vi "Get Software root and experiment.vi"(0 "Application in":refnum<vi>, 1 "This VI":refnum<vi>, 5 "Experiment name in":string, 7 "Sotware root in":string, 9 "FileVersion":string, 11 "error in":errorcluster) -> (3 "Yes?":bool, 4 "Numeric":i32, 6 "Mcast address":string, 10 "Sotware root out":string, 14 "Experiment namet":string, 15 "error out":errorcluster)   [LabVIEW 2020]
doc: "This vi find out experiment from arguments and get software root"
uses:
  Shared/MySQL/Preset Query Enum.ctl
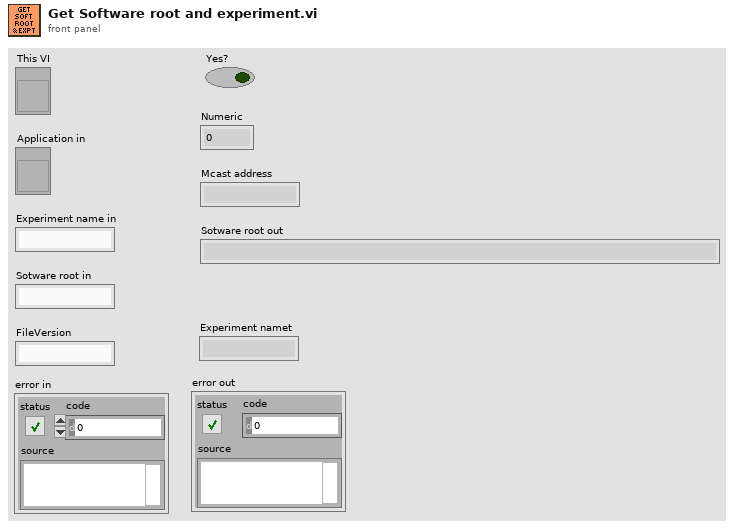
[diagram p1: front panel]
types:
  T1 = typedef "Preset Query Enum.ctl" = enum16{"Get Locations", "Get all IPs and MACs", "Get classes", "Get expt variables to set at scanstart for particular device", "Get expt devices and variables with start values", "Get expt devices and variables (with data to get)", "Get expt devices with data to get", "Get Expt devices and GUIs", "Get all devices basic properties", "Get Virtual Devices Core Info", "Get Expt names", "Get experiment basic properties", "Get experiment alarm variables", "Get MC Ports", "Get device network comm port", "Get devicetype lvclass path", "Get basic device properties", "Get Init Order", "Get all setable variables of a device", "Get device variable aliases", "Get force values of all settable variables", "Get all variables of a devicetype", "Get all variables of a device", "Get plotter details", "Get Saved Scans", "Get Scan Info", "GetGeneralGUIs", "Get expt for plotter", "Get plotter IDs from expt", "Get all devices", "Get all Virtual Devices", "Get all aliases", "Get variable and device info for Virtual Device", "GetItemLocatorIP", "Get IPs for GUIs", "Get DeviceType from Device", "GetLocalPortRange", "GetDevicePresetVariables", "Get Device Configuration", "GetAllPresetNames", "GetAllConfigurationNames", "GetPresetDeviceNames"}
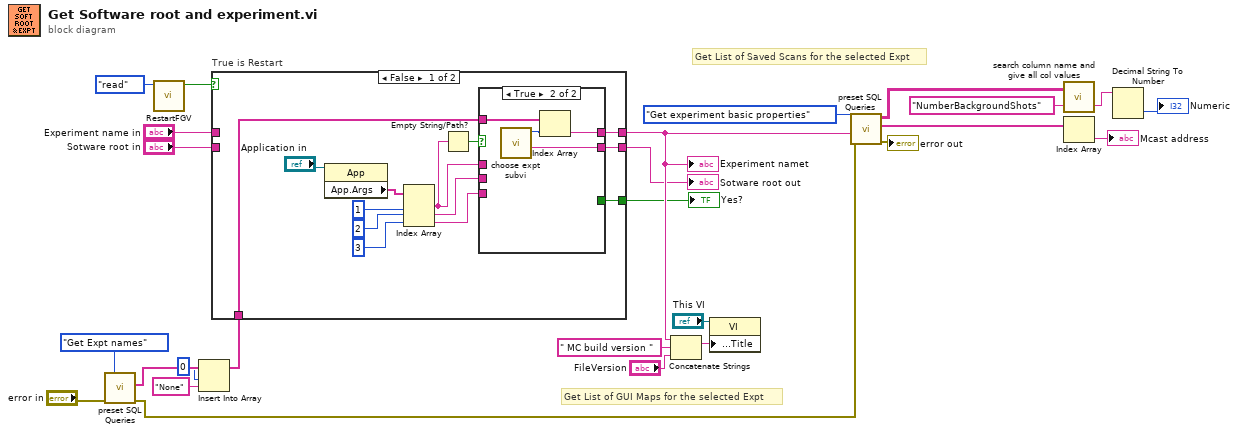
[diagram p0: block diagram]
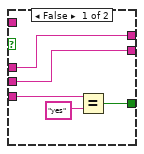
[diagram p2: hidden frame]
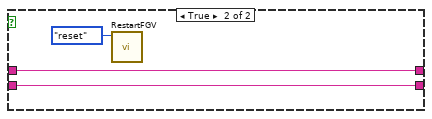
[diagram p3: hidden frame]
diagram:
  # "Get List of Saved Scans for the selected Expt"
  # "Get List of GUI Maps for the selected Expt"
  n1 = call "preset SQL Queries.vi"("error in (no error)"="error in", "Preset Query"=Preset_Query_Enum."Get Expt names") -> ("error out"=w1:errorcluster, "1st column 1st data"=w5:string[])  [unwired: 7 in, 1 out]
  n2 = call "RestartFGV.vi"("Function"=enum16{"set", "reset", "read"}."read") -> ("first call out"=w13:bool)  [unwired: 9 in, 1 out]
  n3 = Insert Into Array(array=w5, index=0, new element="None" ("new element/subarray")) -> (w7:string[])
  n4 = case "True is Restart" shown="False" w13 {
    tunnel: w7 -> [w39 _]
    tunnel: [w38 w50] -> w8
    tunnel: [w37 w51] -> w20
    tunnel: "Experiment name in" -> [_ w51]
    tunnel: "Sotware root in" -> [_ w50]
    tunnel: [w27 _] -> w19
    frame False {
      n5 = property class="App"(reference="Application in") -> ("App.Args"=w34:string[])  [unwired: 1 in, 2 out]
      n6 = Index Array(array=w34, index #1=1 ("index"), index #2=2 ("index"), index #3=3 ("index")) -> (element #1=w30:string, element #2=w31:string, element #3=w28:string)
      n7 = Empty String/Path?(string/path=w30) -> (empty?=w33:bool)
      n8 = case shown="True" w33 {
        tunnel: w39 -> [_ w47]
        tunnel: [w41 w46] -> w38
        tunnel: [w44 w45] -> w37
        tunnel: w31 -> [w41 _]
        tunnel: w30 -> [w44 _]
        tunnel: w28 -> [w40 _]
        tunnel: [w42 _] -> w27
        frame False {
          n9 = Equal?(x=w40, y="yes") -> (x = y?=w42:bool)
        }
        frame True {
          n10 = call "choose expt subvi.vi"() -> ("Software root"=w46:string, "Choosen\nExperiment out"=w48:u16)  [unwired: 10 in]
          n11 = Index Array(array=w47, index=w48) -> (element=w45:string)
        }
      }
    }
    frame True {
      n12 = call "RestartFGV.vi"("Function"=enum16{"set", "reset", "read"}."reset") -> ()  [unwired: 9 in, 2 out]
    }
  }
  "Experiment namet" <- w20
  "Yes?" <- w19
  "Sotware root out" <- w8
  n13 = Concatenate Strings(w20, " MC build version " ("string"), "FileVersion") -> (w16:string)
  n14 = property class="VI"(reference="This VI", "Front Panel.Title"=w16) -> ()  [unwired: 1 in, 2 out]
  n15 = call "preset SQL Queries.vi"("error in (no error)"=w1, "Expt name / MCIP/ Variable/Preset Name"=w20, "Preset Query"=Preset_Query_Enum."Get experiment basic properties") -> ("error out"=→"error out":errorcluster, "1st column 1st data"=w22:string[], "data"=w23:string[][])  [unwired: 6 in]
  n16 = call "search column name and give all col values.vi"("column name to get"="NumberBackgroundShots", "input 2d array"=w23) -> ("First value"=w25:string)  [unwired: 1 out]
  n17 = Index Array(array=w22) -> (element=→"Mcast address":string)  [unwired: 1 in]
  n18 = Decimal String To Number(string=w25) -> (number=→"Numeric":i32)  [unwired: 2 in, 1 out]
